vi "AH_MEAS.vi"(0 "Config Cluster In":T3={"General"={"Config.ini"=path "", "Default Logging Path"=path ""}, "Hardware"={"Measure Rate (1/s)"=0, "HP DMM VISA"="", "LS 335 VISA"="", "HP DM"={"Range"=enum."Autorange", "Autozero"=FALSE, "Display"=enum."3 1/2 Digit", "Blank LCD"=FALSE}}, "Operation"={"Operation Mode"=enum."Logging", "Status"="", "NewLog?"=FALSE, "OvenWarn"=FALSE}}, 5 "Data Cluster In":T1 {"GUI Data Cluster"."SBR" format="%08b"}, 11 "error in (no error)":errorcluster) -> (2 "Cap Ind":string, 3 "Los Ind":string, 4 "Configuration Cluster Out":T3={"General"={"Config.ini"=path "", "Default Logging Path"=path ""}, "Hardware"={"Measure Rate (1/s)"=0, "HP DMM VISA"="", "LS 335 VISA"="", "HP DM"={"Range"=enum."Autorange", "Autozero"=FALSE, "Display"=enum."3 1/2 Digit", "Blank LCD"=FALSE}}, "Operation"={"Operation Mode"=enum."Idle-Off", "Status"="", "NewLog?"=FALSE, "OvenWarn"=FALSE}}, 6 "Data Cluster Out":T1 {"GUI Data Cluster"."SBR" format="%08b"}, 8 "Cap":dbl, 10 "Los":dbl, 13 "Error":i32, 14 "ExVolt":dbl, 15 "error IO":errorcluster)   [LabVIEW 2021]
uses:
  Mode_Enum.ctl
  Config_Cluster.ctl
  Measurement_Cluster.ctl
  Data_Cluster.ctl
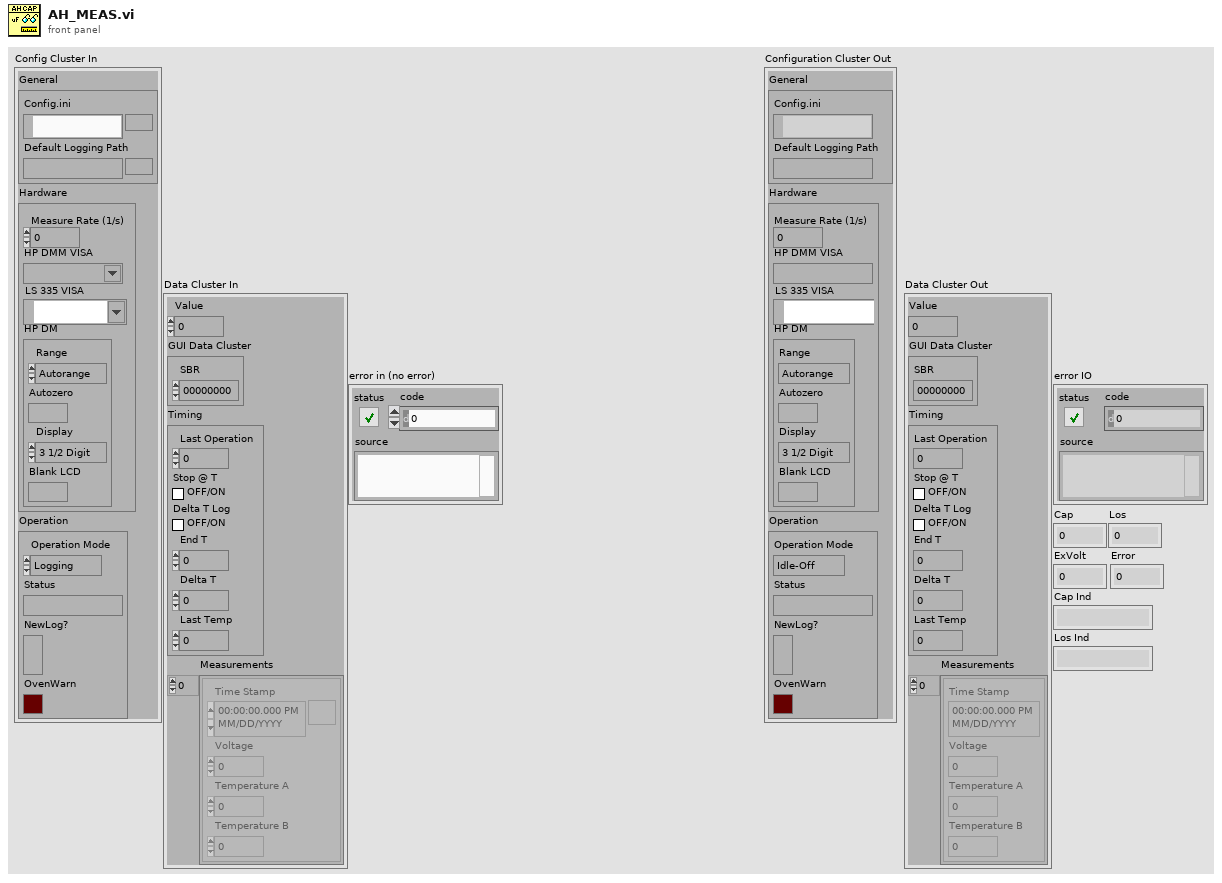
[diagram p1: front panel]
types:
  T1 = typedef "Data_Cluster.ctl" = cluster{"Value":dbl, "GUI Data Cluster":cluster{"SBR":u16}, "Timing":cluster{"Last Operation":dbl, "Stop @ T":bool, "Delta T Log":bool, "End T":dbl, "Delta T":dbl, "Last Temp":dbl}, "Measurements":T2[]}
  T2 = typedef "Measurement_Cluster.ctl" = cluster{"Time Stamp":timestamp, "Voltage":dbl, "Temperature A":dbl, "Temperature B":dbl}
  T3 = typedef "Config_Cluster.ctl" = cluster{"General":cluster{"Config.ini":path, "Default Logging Path":path}, "Hardware":cluster{"Measure Rate (1/s)":i32, "HP DMM VISA":refnum<visa-resource-name>, "LS 335 VISA":refnum<visa-resource-name>, "HP DM":cluster{"Range":enum16{"Autorange", "30mV", "300mV", "3V", "30V"}, "Autozero":bool, "Display":enum16{"3 1/2 Digit", "4 1/2 Digit", "5 1/2 Digit"}, "Blank LCD":bool}}, "Operation":cluster{"Operation Mode":T4, "Status":string, "NewLog?":bool, "OvenWarn":bool}}
  T4 = typedef "Mode_Enum.ctl" = enum16{"OvenNRDY", "Logging", "Idle-Off", "Idle"}
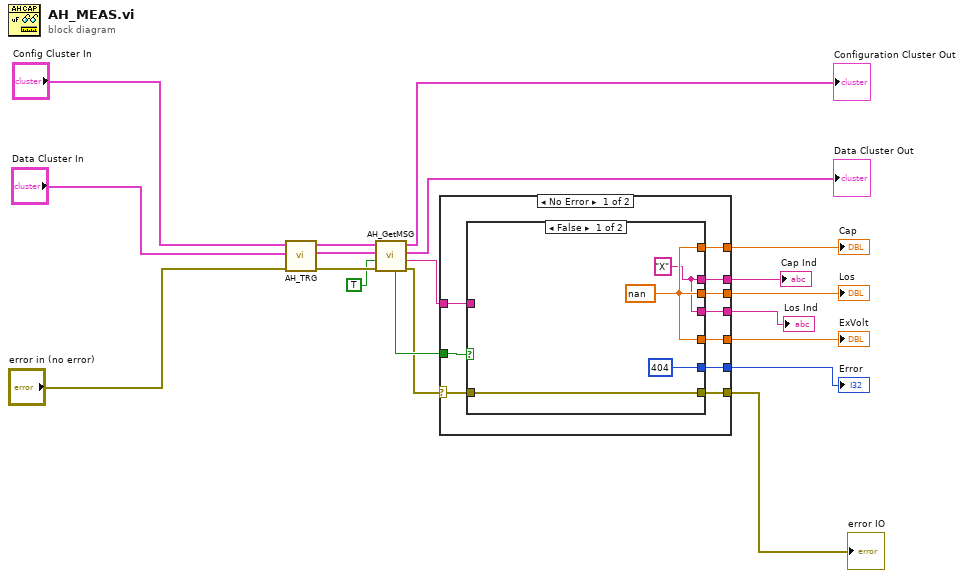
[diagram p0: block diagram]
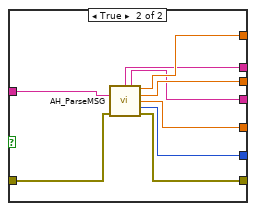
[diagram p2: hidden frame]
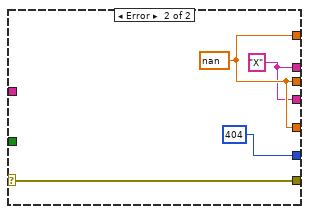
[diagram p3: hidden frame]
diagram:
  n1 = call "AH_TRG.vi"("error in (no error)"="error in (no error)", "Data Cluster In"="Data Cluster In", "Config Cluster In"="Config Cluster In") -> ("error out"=w17:errorcluster, "Data Cluster In Out"=w18:T1, "Config Cluster Out"=w19:T3)  [unwired: 6 in]
  n2 = call "AH_GetMSG.vi"("error in (no error)"=w17, "Halt For RQS"=TRUE, "Data Cluster In"=w18, "Config Cluster In"=w19) -> ("error IO"=w9:errorcluster, "read buffer"=w3:string, "Data Cluster Out"=→"Data Cluster Out":T1, "Configuration Cluster Out"=→"Configuration Cluster Out":T3, "MSG Res"=w10:bool)  [unwired: 2 in, 1 out]
  n3 = case shown="No Error" w9 {
    selector: w9 -> [w28 w44]
    tunnel: w10 -> [w29 _]
    tunnel: [w27 w44] -> w8
    tunnel: [w26 w46] -> w7
    tunnel: [w25 w46] -> w6
    tunnel: [w24 w46] -> w5
    tunnel: [w23 404] -> w4
    tunnel: w3 -> [w22 _]
    tunnel: [w21 w43] -> w2
    tunnel: [w20 w43] -> w1
    frame No Error {
      n4 = case shown="False" w29 {
        tunnel: w28 -> [w33 w37]
        tunnel: [w33 w38] -> w27
        tunnel: [w32 w42] -> w26
        tunnel: [w32 w41] -> w25
        tunnel: [w32 w40] -> w24
        tunnel: [404 w39] -> w23
        tunnel: w22 -> [_ w36]
        tunnel: [w30 w35] -> w21
        tunnel: [w30 w34] -> w20
        frame False {
          w30 = "X" ("Cap Ind")
          w32 = nan
        }
        frame True {
          n5 = call "AH_ParseMSG.vi"("InputMSG"=w36, "error in (no error)"=w37) -> ("Cap Ind"=w35:string, "Los Ind"=w34:string, "Cap"=w42:dbl, "Los"=w41:dbl, "ExVolt"=w40:dbl, "Error"=w39:i32, "error out"=w38:errorcluster)  [unwired: 7 in]
        }
      }
    }
    frame Error {
      w43 = "X" ("Cap Ind")
      w46 = nan
    }
  }
  "error IO" <- w8
  "Cap" <- w7
  "Los" <- w6
  "ExVolt" <- w5
  "Error" <- w4
  "Cap Ind" <- w2
  "Los Ind" <- w1
